vi "glb_DataLog Runtime Parameterisation.vi"() -> ()   [LabVIEW 2012]
panel:
  in  "max string mem":i32=67108864
  in  "current database":path
  in  "min capacity":i32=32
  in  "max points":i32=4194304
  in  "#tags":i32
  in  "recovery directory":path
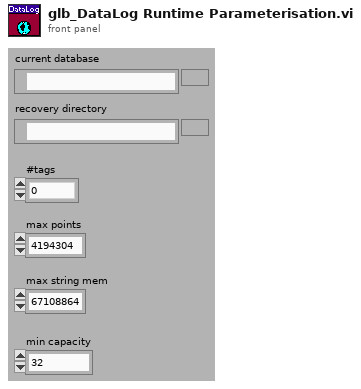
[diagram p1: front panel]
diagram:
